vi "SwerveChooseAngle_Luke.vi"(2 "Hysteresis (deg)":dbl=10.0 format="%#_13g", 3 "Goal Angle (deg)":dbl format="%#_13g", 4 "Current Angle (deg)":dbl format="%#_13g") -> (0 "Invert Speed  Motor (?)":bool, 1 "Angular Distance (deg)":dbl format="%_4g")   [LabVIEW 2019]
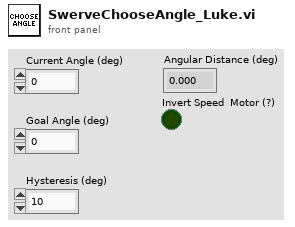
[diagram p1: front panel]
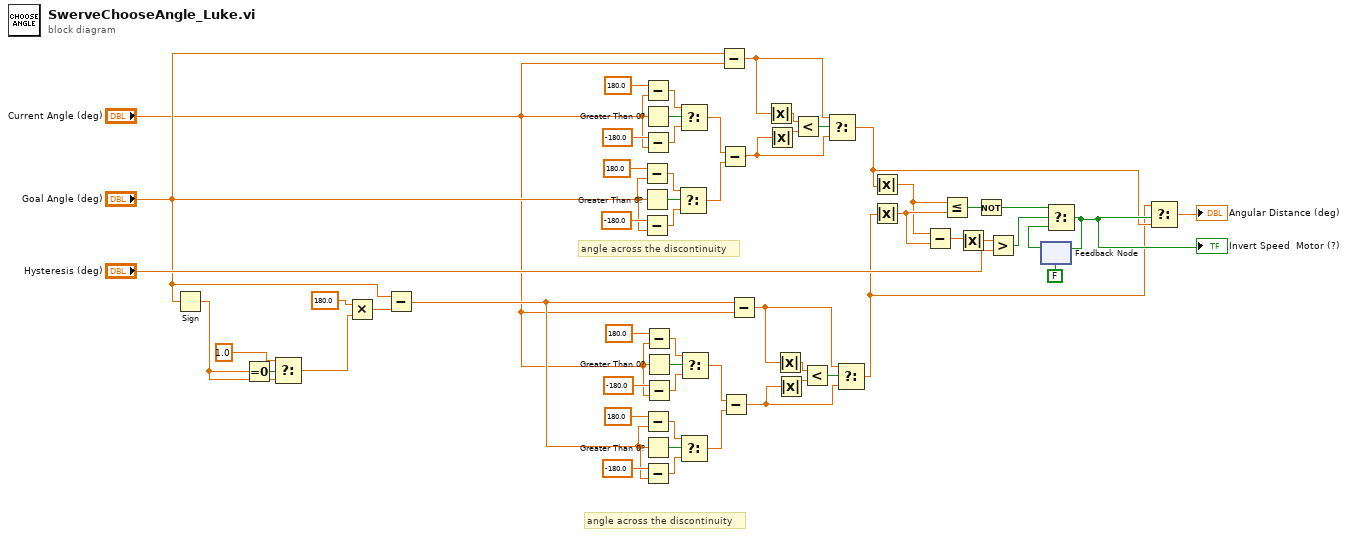
[diagram p0: block diagram]
diagram:
  # "angle across the discontinuity"
  # "angle across the discontinuity"
  n1 = Sign(1:"Goal Angle (deg)") -> (0:w6:dbl)
  n2 = Equal To 0?(x=w6) -> (x = 0?=w7:bool)
  n3 = Select(t=1.0, s=w7, f=w6) -> (s? t:f=w3:dbl)
  n4 = Multiply(x=180.0 ("y"), y=w3) -> (x*y=w57:dbl)
  n5 = Subtract(x="Goal Angle (deg)", y=w57) -> (x-y=w30:dbl)
  n6 = Subtract(x=180.0, y="Goal Angle (deg)") -> (x-y=w18:dbl)
  n7 = Greater Than 0?(x="Goal Angle (deg)") -> (x > 0?=w20:bool)
  n8 = Subtract(x=-180.0, y="Goal Angle (deg)") -> (x-y=w16:dbl)
  n9 = Subtract(x=180.0, y="Current Angle (deg)") -> (x-y=w23:dbl)
  n10 = Greater Than 0?(x="Current Angle (deg)") -> (x > 0?=w25:bool)
  n11 = Subtract(x=-180.0, y="Current Angle (deg)") -> (x-y=w21:dbl)
  n12 = Subtract(x=180.0, y=w30) -> (x-y=w39:dbl)
  n13 = Greater Than 0?(x=w30) -> (x > 0?=w41:bool)
  n14 = Subtract(x=-180.0, y=w30) -> (x-y=w37:dbl)
  n15 = Subtract(x=180.0, y="Current Angle (deg)") -> (x-y=w45:dbl)
  n16 = Greater Than 0?(x="Current Angle (deg)") -> (x > 0?=w47:bool)
  n17 = Subtract(x=-180.0, y="Current Angle (deg)") -> (x-y=w43:dbl)
  n18 = Select(t=w18, s=w20, f=w16) -> (s? t:f=w14:dbl)
  n19 = Select(t=w23, s=w25, f=w21) -> (s? t:f=w15:dbl)
  n20 = Select(t=w39, s=w41, f=w37) -> (s? t:f=w35:dbl)
  n21 = Select(t=w45, s=w47, f=w43) -> (s? t:f=w36:dbl)
  n22 = Subtract(x="Goal Angle (deg)", y="Current Angle (deg)") -> (x-y=w26:dbl)
  n23 = Subtract(x=w15, y=w14) -> (x-y=w11:dbl)
  n24 = Subtract(x=w36, y=w35) -> (x-y=w34:dbl)
  n25 = Subtract(x=w30, y="Current Angle (deg)") -> (x-y=w31:dbl)
  n26 = Absolute Value(x=w26) -> (abs(x)=w27:dbl)
  n27 = Absolute Value(x=w11) -> (abs(x)=w28:dbl)
  n28 = Absolute Value(x=w31) -> (abs(x)=w32:dbl)
  n29 = Absolute Value(x=w34) -> (abs(x)=w33:dbl)
  n30 = Less?(x=w27, y=w28) -> (x < y?=w29:bool)
  n31 = Less?(x=w32, y=w33) -> (x < y?=w42:bool)
  n32 = Select(t=w26, s=w29, f=w11) -> (s? t:f=w2:dbl)
  n33 = Select(t=w31, s=w42, f=w34) -> (s? t:f=w1:dbl)
  n34 = Absolute Value(x=w2) -> (abs(x)=w48:dbl)
  n35 = Absolute Value(x=w1) -> (abs(x)=w49:dbl)
  n36 = Subtract(x=w48, y=w49) -> (x-y=w53:dbl)
  n37 = Less Or Equal?(x=w48, y=w49) -> (x <= y?=w10:bool)
  n38 = Absolute Value(x=w53) -> (abs(x)=w52:dbl)
  n39 = Not(x=w10) -> (.not. x?=w9:bool)
  n40 = Greater?(x=w52, y="Hysteresis (deg)") -> (0:w50:bool)
  n41 = feedback #1(FALSE) -> (w55:bool)
  n42 = Select(t=w9, s=w50, f=w55) -> (s? t:f=w8:bool)
  "Invert Speed  Motor (?)" <- w8
  n43 = feedback-in #1(w8) -> ()
  n44 = Select(t=w1, s=w8, f=w2) -> (s? t:f=→"Angular Distance (deg)":dbl)
